vi "Close.vi"(8 "Error In":errorcluster, 11 "Error Handling In":refnum<class "Error Handling.lvclass">) -> (0 "Error Out":errorcluster)   [LabVIEW 2021, in "Error Handling.lvclass"]
uses:
  Error Handling.lvclass
  Process/Process.lvclass
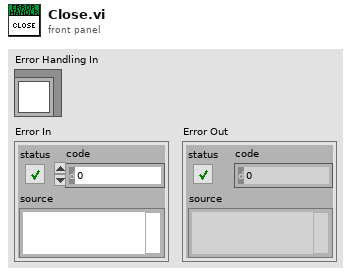
[diagram p1: front panel]
types:
  T1 = typedef "Error Handling.lvclass/Data.ctl" = cluster{"Log File Reference":refnum<file>}
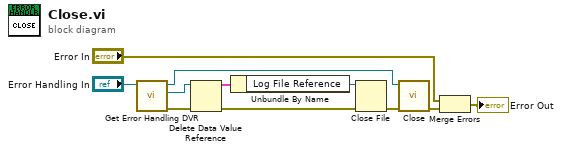
[diagram p0: block diagram]
diagram:
  n1 = call "Get Error Handling DVR.vi"("Error Handling In"="Error Handling In") -> ("Error Out"=w5:errorcluster, "DVR"=w6:refnum<data-value>, "Error Handling Out"=w1:refnum<class "Error Handling.lvclass">)  [unwired: 8 in]
  n2 = Delete Data Value Reference(data value reference=w6, error in=w5) -> (data value=w8:T1, error out=w3:errorcluster)
  n3 = Unbundle By Name(w8) -> ("Log File Reference"=w4:refnum<file>)
  n4 = Close File(refnum=w4, error in=w3) -> (error out=w2:errorcluster)  [unwired: 1 out]
  n5 = call-parent "Close.vi"("Error In"=w2, "Process In"=w1) -> ("Error Out"=w11:errorcluster)  [unwired: 9 in]
  n6 = Merge Errors("Error In", w11) -> (→"Error Out":errorcluster)
